vi "execution class name.vi"(8 "error in":errorcluster, 11 "configuration in":refnum<class "testmod configuration.lvclass">) -> (0 "error out":errorcluster, 2 "execution class":string, 3 "configuration out":refnum<class "testmod configuration.lvclass">)   [LabVIEW 2013, in "testmod configuration.lvclass"]
uses:
  testmod configuration.lvclass
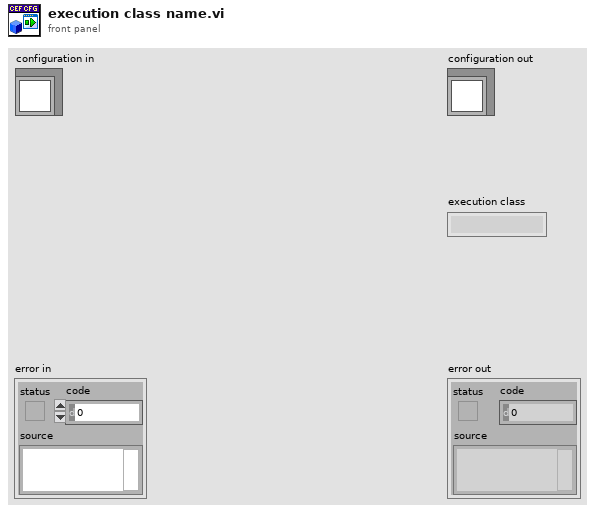
[diagram p1: front panel]
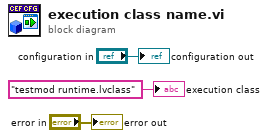
[diagram p0: block diagram]
diagram:
  "error out" <- "error in"
  "configuration out" <- "configuration in"
  "execution class" <- "testmod runtime.lvclass" ("execution class")
